vi "OAT Output Trigger Event.vi"   [LabVIEW 2017, in "SoundVib_OAUtility.lvlib"]
doc: "Detects the first level-crossing condition. The <B>upper setpoint</B> and <B>lower setpoint</B> of the threshold and the <B>hysteresis</B> specify the trigger conditions. Wire data to the <B>signal in</B> input to determine the polymorphic instance to use or manually select the instance."
uses:
  <vilib>/addons/Sound and Vibration/Order Analysis/Utility/SoundVib_OAUtility.lvlib
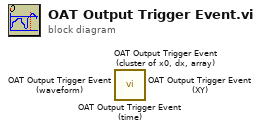
[diagram p0: block diagram]
diagram:
  n1 = call <vilib>:"OAT Output Trigger Event (time).vi"() -> ()  [unwired: 14 in, 2 out]
  n2 = call <vilib>:"OAT Output Trigger Event (cluster of x0, dx, array).vi"() -> ()  [unwired: 14 in, 2 out]
  n3 = call <vilib>:"OAT Output Trigger Event (waveform).vi"() -> ()  [unwired: 14 in, 2 out]
  n4 = call <vilib>:"OAT Output Trigger Event (XY).vi"() -> ()  [unwired: 14 in, 2 out]
